vi "14_20_Fxp_addation.vi"(1 "y":fxp<+/-,20,14>, 2 "x":fxp<+/-,20,14>) -> (0 "x+y":fxp<+/-,21,15> format="%.41g")   [LabVIEW 2020]
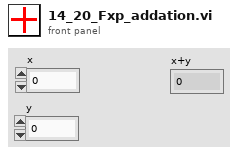
[diagram p1: front panel]
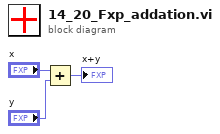
[diagram p0: block diagram]
diagram:
  n1 = Add(x="x", y="y") -> (x+y=→"x+y":fxp<+/-,21,15>)
